vi "RecoverControls.vi"(4 "Variable":string[](array[string])=["Center"], 6 "Control":string[](array[string])=["Center Voltage"], 8 "Name":string, 9 "Value":variant, 10 "Pages":refnum<vi>[](array[refnum]), 11 "reference":refnum<vi>) -> ()   [LabVIEW 2013]
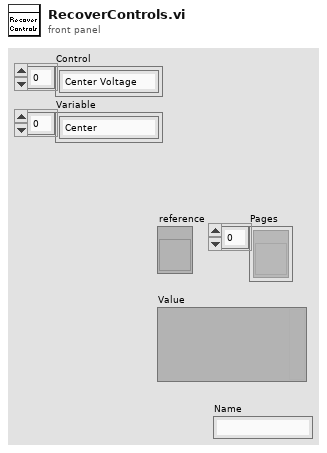
[diagram p1: front panel]
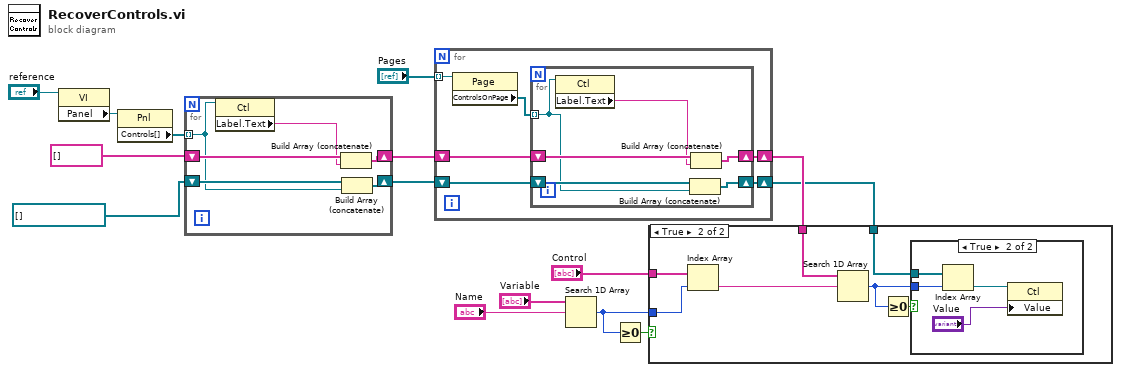
[diagram p0: block diagram]
diagram:
  n1 = property class="VI"(reference="reference") -> ("Panel"=w12:refnum<vi>)  [unwired: 1 in, 2 out]
  n2 = property class="Pnl"(reference=w12) -> ("Controls[]"=w13:refnum<vi>[])  [unwired: 1 in, 2 out]
  n3 = for {
    tunnel: w13 -> [w16] mode=indexing
    shift-right: [w20] -> w14
    shift-left: string[] [] -> [w21]
    shift-right: [w19] -> w3
    shift-left: refnum<vi>[] [] -> [w18]
    n4 = property class="Ctl"(reference=w16) -> ("Label.Text"=w17:string)  [unwired: 1 in, 2 out]
    n5 = Build Array (concatenate)(w21, w17) -> (w20:string[])
    n6 = Build Array (concatenate)(w18, w16) -> (w19:refnum<vi>[])
  }
  n7 = for {
    shift-right: [w26] -> w2
    shift-left: w14 -> [w27]
    tunnel: "Pages" -> [w25] mode=indexing
    shift-right: [w23] -> w1
    shift-left: w3 -> [w22]
    n8 = property class="Page"(reference=w25) -> ("ControlsOnPage"=w24:refnum<vi>[])  [unwired: 1 in, 2 out]
    n9 = for {
      shift-right: [w33] -> w26
      shift-left: w27 -> [w32]
      tunnel: w24 -> [w28] mode=indexing
      shift-right: [w30] -> w23
      shift-left: w22 -> [w31]
      n10 = property class="Ctl"(reference=w28) -> ("Label.Text"=w29:string)  [unwired: 1 in, 2 out]
      n11 = Build Array (concatenate)(w31, w28) -> (w30:refnum<vi>[])
      n12 = Build Array (concatenate)(w32, w29) -> (w33:string[])
    }
  }
  n13 = Search 1D Array(1D array="Variable", element="Name") -> (index of element=w6:i32)  [unwired: 1 in]
  n14 = Greater Or Equal To 0?(x=w6) -> (x >= 0?=w8:bool)
  n15 = case shown="True" w8 {
    tunnel: "Control" -> [_ w40]
    tunnel: w6 -> [_ w39]
    tunnel: w2 -> [_ w38]
    tunnel: w1 -> [_ w35]
    frame False {
    }
    frame True {
      n16 = Index Array(array=w40, index=w39) -> (element=w37:string)
      n17 = Search 1D Array(1D array=w38, element=w37) -> (index of element=w34:i32)  [unwired: 1 in]
      n18 = Greater Or Equal To 0?(x=w34) -> (x >= 0?=w36:bool)
      n19 = case shown="True" w36 {
        tunnel: w35 -> [_ w44]
        tunnel: w34 -> [_ w43]
        frame False {
        }
        frame True {
          n20 = Index Array(array=w44, index=w43) -> (element=w42:refnum<vi>)
          n21 = property class="Ctl"(reference=w42, "Value"="Value") -> ()  [unwired: 1 in, 2 out]
        }
      }
    }
  }
